vi "WritePanelData_test_ringsvaluecorrect.vi"(8 "error in (no error)":errorcluster, 11 "Maui.Test.DefaultDirectory in":refnum<class "Maui.Test.DefaultDirectory.lvclass">) -> (0 "error out":errorcluster, 3 "Maui.Test.DefaultDirectory out":refnum<class "Maui.Test.DefaultDirectory.lvclass">)   [LabVIEW 2020, in "Maui.Test.DefaultDirectory.lvclass"]
uses:
  Maui.Test.DefaultDirectory.lvclass
  Maui.Test.DefaultDirectory.lvclass/Maui.Test.DefaultDirectory.ctl
  <vilib>/addons/_JKI Toolkits/Caraya/classes/Assert/Assert Equal Value_Variant.vi
  <vilib>/addons/_JKI Toolkits/Caraya/classes/Test/Test.lvclass
  <vilib>/addons/_JKI Toolkits/Caraya/classes/Assert/Assert.lvclass
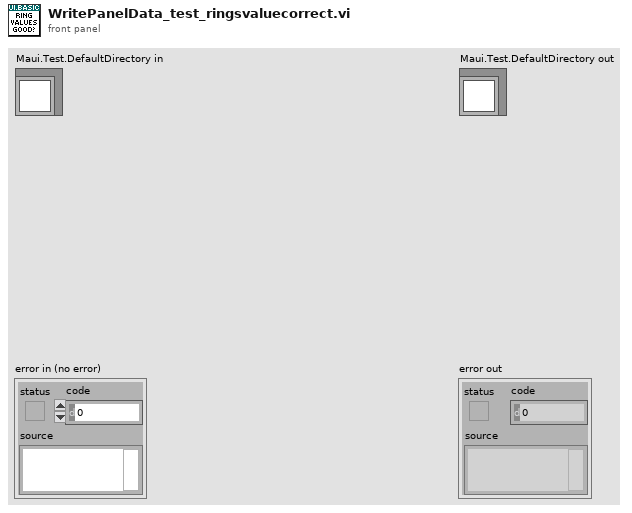
[diagram p1: front panel]
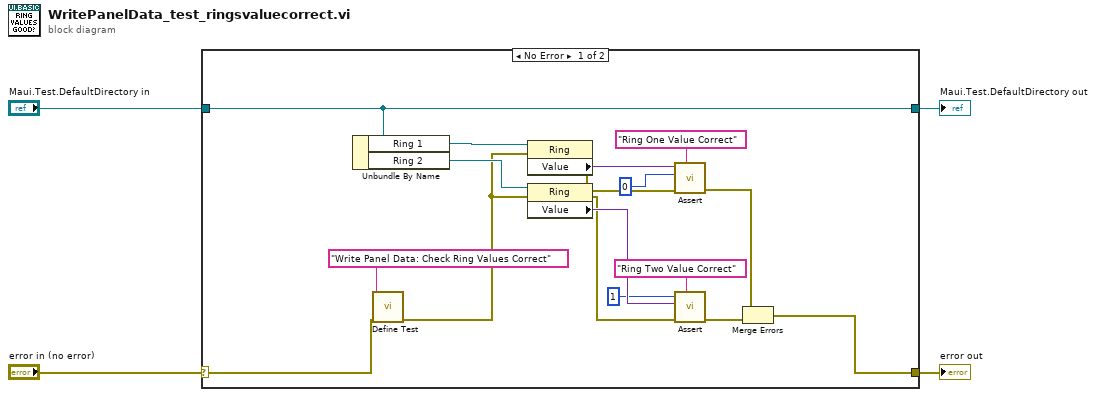
[diagram p0: block diagram]
diagram:
  n1 = case shown="No Error" "error in (no error)" {
    selector: "error in (no error)" -> [w18 w23]
    tunnel: [w17 w23] -> w3
    tunnel: [w21 w22] -> w1
    tunnel: "Maui.Test.DefaultDirectory in" -> [w21 w22]
    frame No Error {
      n2 = Unbundle By Name(w21) -> ("Ring 1"=w15:refnum<vi>, "Ring 2"=w13:refnum<vi>)
      n3 = call <vilib>:"Define Test.vi"("error in (no error)"=w18, "Label (VI Title)"="Write Panel Data: Check Ring Values Correct") -> ("error out"=w7:errorcluster)  [unwired: 9 in]
      n4 = property on="Property Node" class="Ring"(reference=w15, error in=w7) -> (error out=w8:errorcluster, "Value"=w14:variant)  [unwired: 1 out]
      n5 = property on="Property Node" class="Ring"(reference=w13, error in=w7) -> (error out=w6:errorcluster, "Value"=w12:variant)  [unwired: 1 out]
      n6 = call-poly <vilib>:"Assert.vi"("Label"="Ring One Value Correct" ("Label (VI Title)"), "error in (no error)"=w8, "Y"=0, "X"=w14) -> ("error out"=w9:errorcluster)  [unwired: 7 in]
      n7 = call-poly <vilib>:"Assert.vi"("Label"="Ring Two Value Correct" ("Label (VI Title)"), "error in (no error)"=w6, "Y"=w12, "X"=1) -> ("error out"=w19:errorcluster)  [unwired: 7 in]
      n8 = Merge Errors(w9, w19) -> (w17:errorcluster)
    }
    frame Error {
    }
  }
  "error out" <- w3
  "Maui.Test.DefaultDirectory out" <- w1
